vi "String to Number no comma.vi"(11 "Number String":string) -> (3 "Numeric":i32)   [LabVIEW 2021]
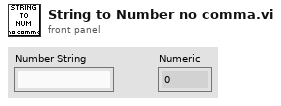
[diagram p1: front panel]
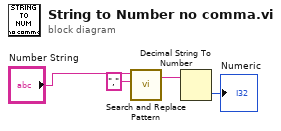
[diagram p0: block diagram]
diagram:
  n1 = call <vilib>:"Search and Replace Pattern.vi"("string"="Number String", "regular expression (\"\")"="," ("regular expression (\"\")")) -> ("result string"=w3:string)  [unwired: 3 in, 1 out]
  n2 = Decimal String To Number(string=w3) -> (number=→"Numeric":i32)  [unwired: 2 in, 1 out]
